vi "get source name.vi"(8 "error in":errorcluster, 11 "timing source in":refnum<class "ms timing source.lvclass">) -> (0 "error out":errorcluster, 2 "source name":string, 3 "timing source out":refnum<class "ms timing source.lvclass">)   [LabVIEW 2013, in "ms timing source.lvclass"]
doc: "Returns the name of the timing source to be used as part of the configuration of a timed loop. For example, the 1 ms timer would return the string \"1 kHz\"."
uses:
  ms timing source.lvclass
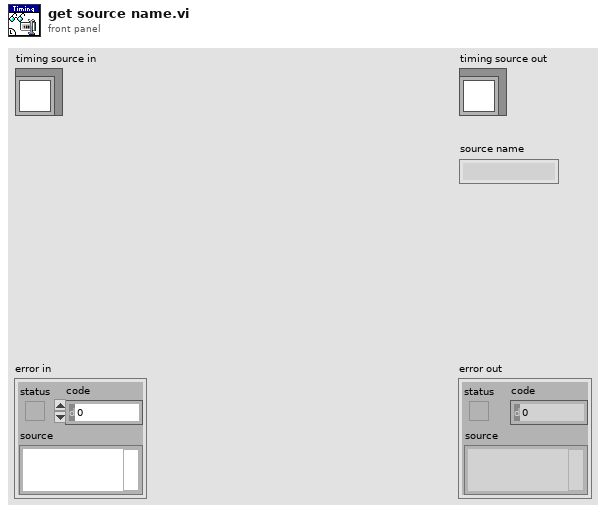
[diagram p1: front panel]
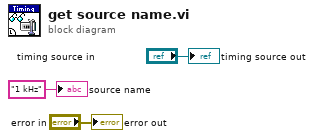
[diagram p0: block diagram]
diagram:
  "error out" <- "error in"
  "timing source out" <- "timing source in"
  "source name" <- "1 kHz" ("source name")
